vi "addSensors.vi"(8 "error in (no error)":errorcluster, 10 "Sensor.lvclass":refnum<class "Sensor.lvclass">, 11 "Tank in":refnum<class "Tank.lvclass">) -> (0 "error out":errorcluster, 3 "Tank out":refnum<class "Tank.lvclass">)   [LabVIEW 2017, in "Tank.lvclass"]
uses:
  Tank.lvclass
  Sensor Class/Sensor.lvclass
  Tank.lvclass/Tank.ctl
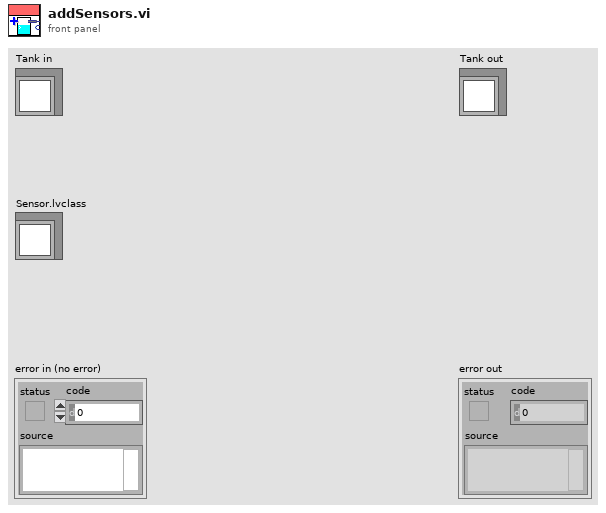
[diagram p1: front panel]
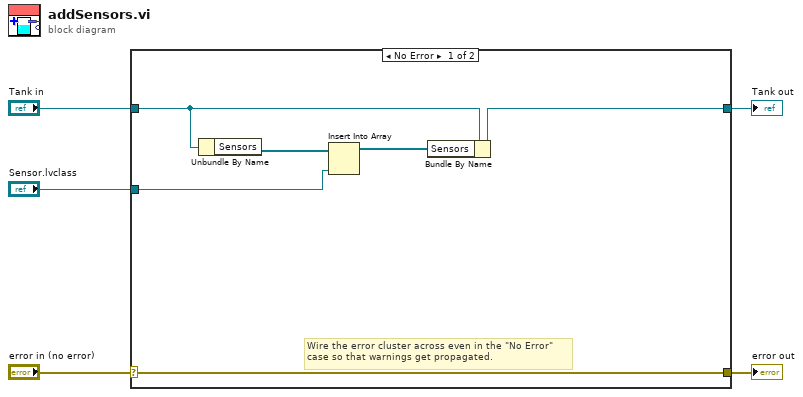
[diagram p0: block diagram]
diagram:
  n1 = case shown="No Error" "error in (no error)" {
    selector: "error in (no error)" -> [w11 w13]
    tunnel: [w11 w13] -> w4
    tunnel: [w9 w12] -> w2
    tunnel: "Tank in" -> [w10 w12]
    tunnel: "Sensor.lvclass" -> [w6 _]
    frame No Error {
      # "Wire the error cluster across even in the \"No Error\"\ncase so that warnings get propagated."
      n2 = Unbundle By Name(w10) -> ("Sensors"=w8:refnum<class "Sensor.lvclass">[])
      n3 = Insert Into Array(array=w8, new element=w6) -> (w7:refnum<class "Sensor.lvclass">[])  [unwired: 1 in]
      n4 = Bundle By Name(cluster=w10, "Sensors"=w7) -> (w9:refnum<class "Tank.lvclass">)
    }
    frame Error {
    }
  }
  "error out" <- w4
  "Tank out" <- w2
